vi "show calibration.vi"(6 "error in":errorcluster, 9 "KCubeDCServo":refnum<k24>) -> (0 "error out":errorcluster, 1 "Power (W)":dbl[](array[numeric]), 2 "Angle (degrees)":dbl[](array[numeric]), 3 "best fit parameters":dbl[](array[numeric]))   [LabVIEW 2023, in "Thorlabs Polarizer.lvlib"]
uses:
  Thorlabs Polarizer.lvlib
  C:/FlashGordon/Development/dll/ThorLabs.MotionControl.KCube.DCServoCLI.dll
  dll/ThorLabs.MotionControl.KCube.DCServoCLI.dll
  Resources/GLOBAL/GLOBAL Time-critical.vi
  polarizer model.vi
  <vilib>/gmath/NumericalOptimization/Nonlinear Curve Fit LM.vi
  <vilib>/gmath/NI_Gmath.lvlib
  Power Meter/Power Meter.lvlib
panel:
  out "Progress":u8(slide) scale=0.0..100.0
  out "XY Graph":cluster{dbl[], dbl[]}[](graph)
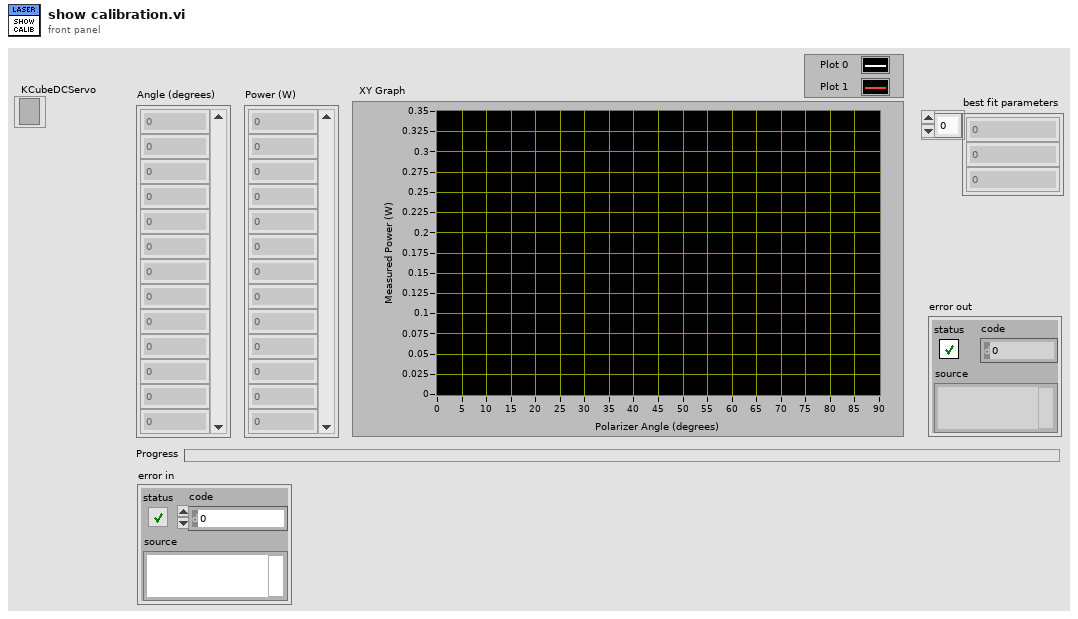
[diagram p1: front panel]
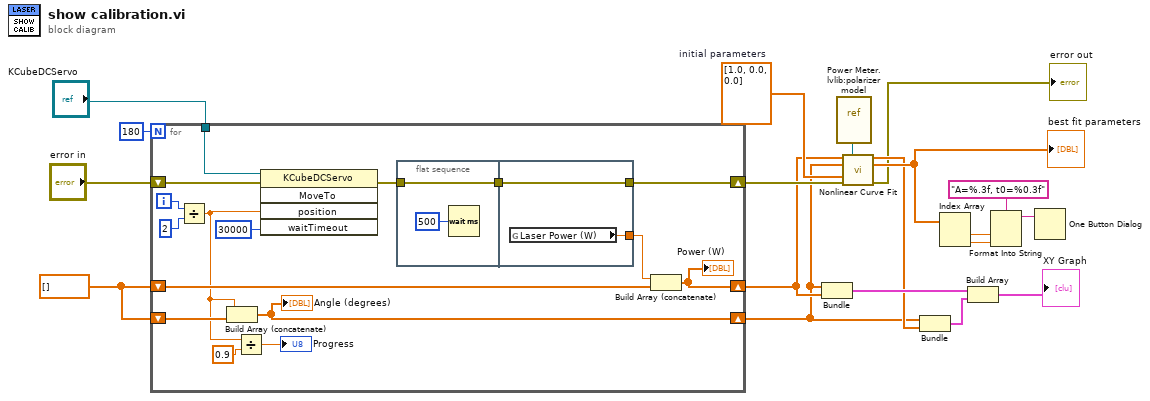
[diagram p0: block diagram]
diagram:
  w7 = dbl[] []
  w10 = dbl[] [1.0, 0.0, 0.0]  # initial parameters
  n1 = for {
    N: 180 -> [_]
    tunnel: "KCubeDCServo" -> [w34]
    shift-right: [w29] -> w4
    shift-left: "error in" -> [w33]
    shift-right: [w25] -> w2
    shift-left: w7 -> [w26]
    shift-right: [w24] -> w1
    shift-left: w7 -> [w21]
    i -> [w31]
    n2 = Divide(x=w31, y=2) -> (x/y=w20:dbl)
    n3 = Build Array (concatenate)(w20, w21) -> (w24:dbl[])
    "Angle (degrees)" <- w24
    n4 = Divide(x=w20, y=0.9) -> (x/y=→"Progress":dbl)
    n5 = invoke class="KCubeDCServo" method="MoveTo"(reference=w34, error in=w33, "position"=w20, "waitTimeout"=30000) -> (error out=w30:errorcluster)  [unwired: 1 in, 4 out]
    n6 = flat-sequence {
      tunnel: w30 -> [w37]
      tunnel: [w37] -> w28
      tunnel: [w39] -> w27
      tunnel: [w38] -> w29
      tunnel: w28 -> [w38]
      frame #0 {
        n7 = Wait (ms)(milliseconds to wait=u32 500) -> ()  [unwired: 1 out]
      }
      frame #1 {
        n8 = global read "GLOBAL Time-critical.vi" "Laser Power (W)"() -> (w39:dbl)
      }
    }
    n9 = Build Array (concatenate)(w27, w26) -> (w25:dbl[])
    "Power (W)" <- w25
  }
  n10 = Bundle(w1, w2) -> (w14:cluster{dbl[], dbl[]})  [unwired: 1 in]
  n11 = vi-ref "Power Meter.lvlib:polarizer model.vi"() -> (w9:refnum<vi>)
  n12 = call-poly <vilib>:"Nonlinear Curve Fit.vi"("Y"=w2, "f(x,a)"=w9, "X"=w1, "initial parameters"=w10, "error in (no error)"=w4) -> ("best nonlinear fit"=w11:dbl[], "best fit parameters"=w17:dbl[], "error out"=→"error out":errorcluster)  [unwired: 5 in, 3 out]
  "best fit parameters" <- w17
  n13 = Bundle(w1, "best nonlinear fit"=w11) -> (w12:cluster{dbl[], "best nonlinear fit":dbl[]})  [unwired: 1 in]
  n14 = Index Array(array=w17) -> (element #1=w16:dbl, element #2=w15:dbl)  [unwired: 2 in]
  n15 = Build Array(w14, w12) -> (→"XY Graph":cluster{dbl[], "best nonlinear fit":dbl[]}[])
  n16 = Format Into String(format string="A=%.3f, t0=%0.3f", w16, w15) -> (resulting string=w19:string)  [unwired: 2 in, 1 out]
  n17 = One Button Dialog(message=w19) -> ()  [unwired: 1 in, 1 out]
